vi "Set Main Properties.vi"(8 "error in (no error)":errorcluster, 10 "Main Page Parameters":T1={"AI Channels Used"=0, "AO Channels Used"=0, "Select channel type to add"="", "Device Name in Max"="PXI1Slot2", "PCL Decimation"=0, "Async Timeout (ms)"=0}, 11 "Ref in":T2 format="%.0x") -> (0 "error out":errorcluster, 3 "Ref out":T2 format="%.0x")   [LabVIEW 2021, in "DAQ Analog InOut System Explorer.lvlib"]
uses:
  DAQ Analog InOut System Explorer.lvlib
  <vilib>/NI VeriStand/Custom Device API/Custom Device Item Ref.ctl
  Types/Main Page Parameters.ctl
  Shared/Constants.vi
  <vilib>/NI VeriStand/Custom Device API/Set Item Property (Variant).vi
  <vilib>/NI VeriStand/Custom Device API/Custom Device API.lvlib
  Shared/DAQ Analog InOut Shared.lvlib
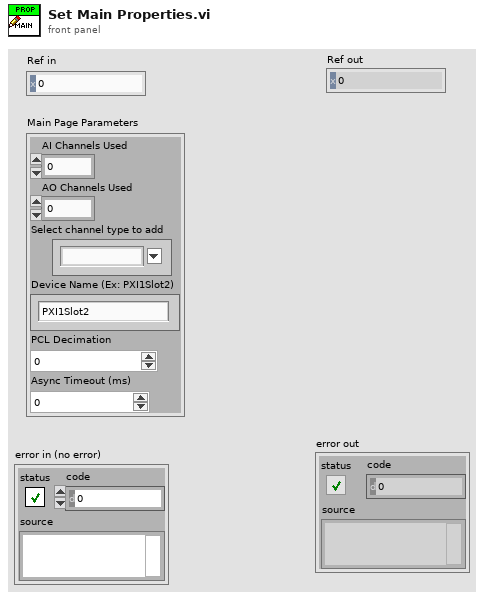
[diagram p1: front panel]
types:
  T1 = typedef "DAQ Analog InOut System Explorer.lvlib/Main Page Parameters.ctl" = cluster{"AI Channels Used":u8, "AO Channels Used":u8, "Select channel type to add":string, "Device Name in Max":string, "PCL Decimation":u16, "Async Timeout (ms)":u16}
  T2 = typedef "Custom Device API.lvlib/Custom Device Item Ref.ctl" = u64
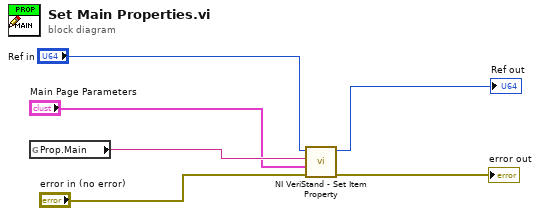
[diagram p0: block diagram]
diagram:
  n1 = global read "Constants.vi" "Prop.Main"() -> (w2:string)
  n2 = call-poly <vilib>:"NI VeriStand - Set Item Property.vi"("error in (no error)"="error in (no error)", "Value"="Main Page Parameters", "Property Name"=w2, "Item Ref in"="Ref in") -> ("error out"=→"error out":errorcluster, "Item Ref out"=→"Ref out":T2)  [unwired: 5 in, 1 out]
